vi "Record Assertion Result.vi"(9 "Test Result":refnum<class "Assertion Result.lvclass">, 10 "Test Method":string, 11 "Test Case Result in":refnum<class "Test Case Result.lvclass">) -> (3 "Test Case Result out":refnum<class "Test Case Result.lvclass">)   [LabVIEW 2020, in "Test Case Result.lvclass"]
uses:
  Test Case Result.lvclass
  Method Result/Method Result.lvclass
  <vilib>/Utility/miscctls.llb/LVMapReplaceAction.ctl
  Assertion Result/Assertion Result.lvclass
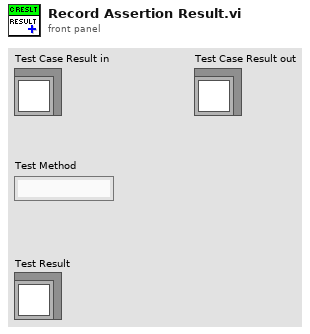
[diagram p1: front panel]
types:
  T1 = typedef "LVMapReplaceAction.ctl" = enum32{"Modify Entry only if found", "Add or Modify Entry", "Delete Entry"}
  T2 = map{string, refnum<class "Method Result.lvclass">}
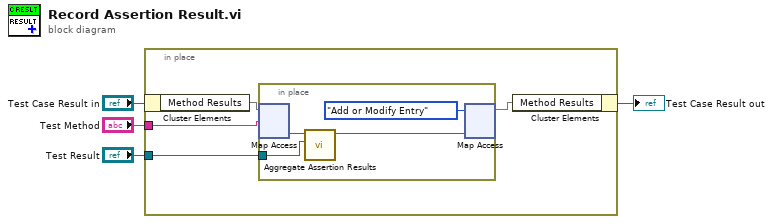
[diagram p0: block diagram]
diagram:
  n1 = in-place {
    in-place-border: "Test Method" -> [w7]
    in-place-border: "Test Result" -> [w6]
    n2 = in-place-cluster #1("Test Case Result in") -> ("Method Results"=w8:T2)
    n3 = in-place {
      in-place-border: w6 -> [w10]
      n4 = in-place-map #2(w8, w7) -> (w12:refnum<class "Method Result.lvclass">)  [unwired: 1 in, 1 out]
      n5 = call "Aggregate Assertion Results.vi"("Assertion Result"=w10, "Method Result In"=w12) -> ("Method Result Out"=w11:refnum<class "Method Result.lvclass">)  [unwired: 9 in]
      n6 = in-place-map #2(w11, LVMapReplaceAction."Add or Modify Entry" ("action")) -> (w5:T2)  [unwired: 2 out]
    }
    n7 = in-place-cluster #1("Method Results"=w5) -> (→"Test Case Result out":refnum<class "Test Case Result.lvclass">)
  }
